vi "Close_ESP.vi"(8 "error in (no error)":errorcluster, 11 "VISA resource name":refnum<visa-resource-name>) -> (0 "error out":errorcluster)   [LabVIEW 2025]
doc: "Cierra la comunicacion del VI con la ESP32\nSiempre debe colocarse al final y afuera de cualquier ciclo para evitar cierres innecesarios"
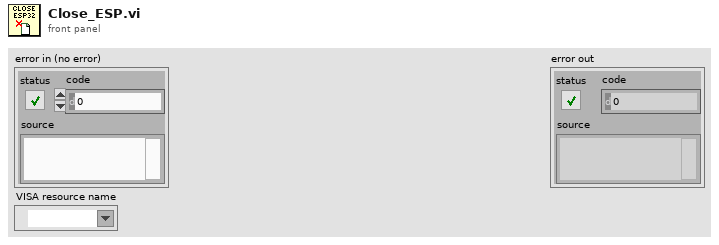
[diagram p1: front panel]
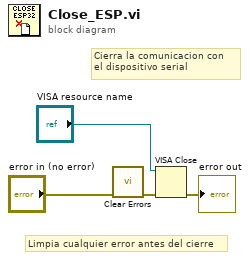
[diagram p0: block diagram]
diagram:
  # "Limpia cualquier error antes del cierre"
  # "Cierra la comunicacion con\nel dispositivo serial"
  n1 = call <vilib>:"Clear Errors.vi"("error in (no error)"="error in (no error)") -> ("error out"=w1:errorcluster)  [unwired: 5 in, 1 out]
  n2 = VISA Close(VISA resource name="VISA resource name", error in (no error)=w1) -> (error out=→"error out":errorcluster)
